vi "magnet_controller.vi"(1 "Arguments":string, 2 "Command":T1(ring)=enum."Hold", 3 "Direction":enum16{"X", "Y", "Z"}(ring)=enum."Y") -> (0 "Response":string)   [LabVIEW 2021]
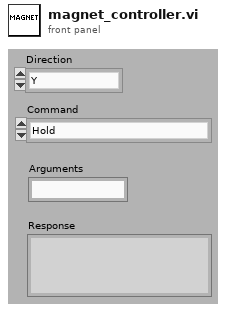
[diagram p1: front panel]
types:
  T1 = enum16{"Read State", "Hold", "Ramp to Set", "Ramp to Zero", "Read Switch Heater", "Switch Heater On", "Switch Heater Off", "Read Voltage", "Read Current", "Read Field", "Read Persistent Field", "Read Target Field", "Set Target Field", "Read Ramp Rate", "Set Ramp Rate"}
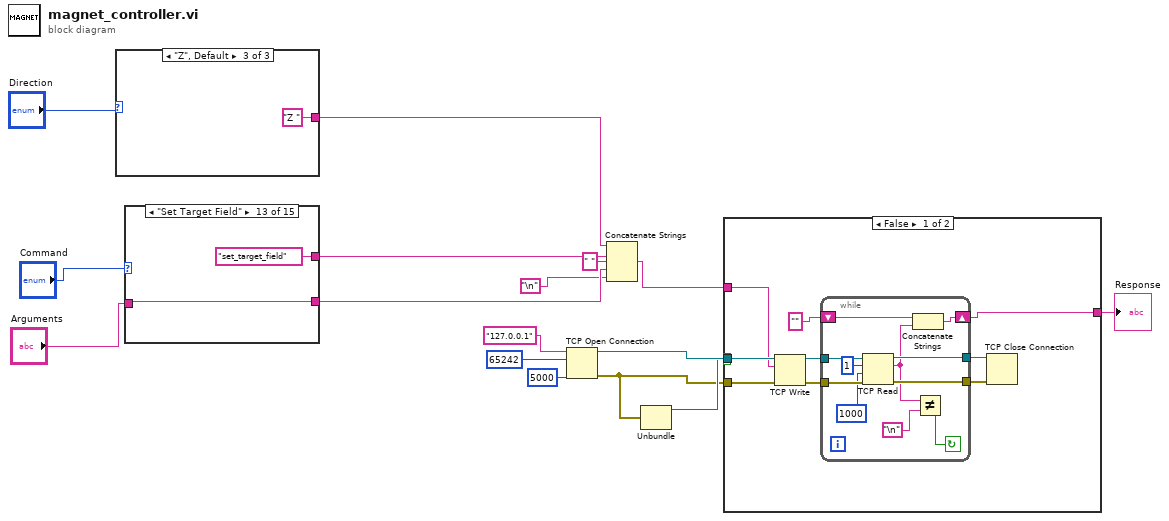
[diagram p0: block diagram]
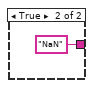
[diagram p2: hidden frame]
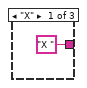
[diagram p3: hidden frame]
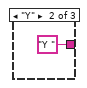
[diagram p4: hidden frame]
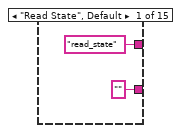
[diagram p5: hidden frame]
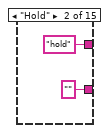
[diagram p6: hidden frame]
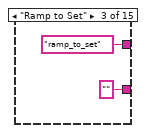
[diagram p7: hidden frame]
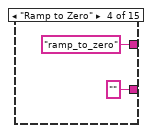
[diagram p8: hidden frame]
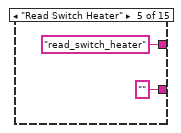
[diagram p9: hidden frame]
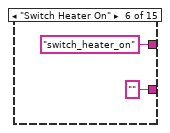
[diagram p10: hidden frame]
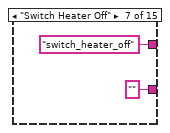
[diagram p11: hidden frame]
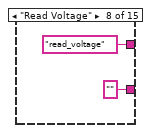
[diagram p12: hidden frame]
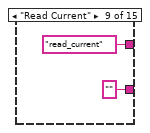
[diagram p13: hidden frame]
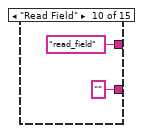
[diagram p14: hidden frame]
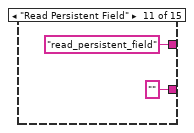
[diagram p15: hidden frame]
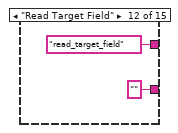
[diagram p16: hidden frame]
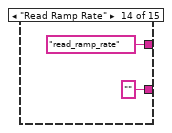
[diagram p17: hidden frame]
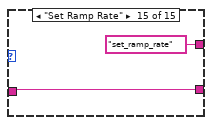
[diagram p18: hidden frame]
diagram:
  n1 = case shown="\"Z\", Default" "Direction" {
    tunnel: ["X " ("string") "Y " ("string") "Z " ("string")] -> w5
    frame "X" {
    }
    frame "Y" {
    }
    frame "Z", Default {
    }
  }
  n2 = case shown="\"Set Target Field\"" "Command" {
    tunnel: ["read_state" ("data in") "hold" ("data in") "ramp_to_set" ("data in") "ramp_to_zero" ("data in") "read_switch_heater" ("data in") "switch_heater_on" ("data in") "switch_heater_off" ("data in") "read_voltage" ("data in") "read_current" ("data in") "read_field" ("data in") "read_persistent_field" ("data in") "read_target_field" ("data in") "set_target_field" ("data in") "read_ramp_rate" ("data in") "set_ramp_rate" ("data in")] -> w12
    tunnel: ["" ("Arguments") "" ("Arguments") "" ("Arguments") "" ("Arguments") "" ("Arguments") "" ("Arguments") "" ("Arguments") "" ("Arguments") "" ("Arguments") "" ("Arguments") "" ("Arguments") "" ("Arguments") w44 "" ("Arguments") w48] -> w9
    tunnel: "Arguments" -> [_ _ _ _ _ _ _ _ _ _ _ _ w44 _ w48]
    frame "Read State", Default {
    }
    frame "Hold" {
    }
    frame "Ramp to Set" {
    }
    frame "Ramp to Zero" {
    }
    frame "Read Switch Heater" {
    }
    frame "Switch Heater On" {
    }
    frame "Switch Heater Off" {
    }
    frame "Read Voltage" {
    }
    frame "Read Current" {
    }
    frame "Read Field" {
    }
    frame "Read Persistent Field" {
    }
    frame "Read Target Field" {
    }
    frame "Set Target Field" {
    }
    frame "Read Ramp Rate" {
    }
    frame "Set Ramp Rate" {
    }
  }
  n3 = TCP Open Connection(address="127.0.0.1", remote port or service name=u16 65242, timeout ms (60000)=5000) -> (connection ID=w14:refnum<k5>, error out=w2:errorcluster)  [unwired: 2 in]
  n4 = Concatenate Strings(w5, w12, " " ("string"), w9, "\n") -> (w13:string)
  n5 = Unbundle(w2) -> ("status"=w3:bool)  [unwired: 2 out]
  n6 = case shown="False" w3 {
    tunnel: w14 -> [w58 _]
    tunnel: w2 -> [w57 _]
    tunnel: w13 -> [w51 _]
    tunnel: [w50 "NaN" ("string")] -> w4
    frame False {
      n7 = TCP Write(connection ID=w58, data in=w51, error in (no error)=w57) -> (connection ID out=w55:refnum<k5>, error out=w56:errorcluster)  [unwired: 1 in, 1 out]
      n8 = while {
        tunnel: w56 -> [w69]
        tunnel: w55 -> [w68]
        tunnel: [w67] -> w54
        tunnel: [w66] -> w53
        shift-right: [w62] -> w50
        shift-left: "" ("string") -> [w63]
        stop <- w61 continue-if-true
        n9 = TCP Read(connection ID=w68, bytes to read=1, error in (no error)=w69, 9:1000 ("timeout ms (25000)")) -> (connection ID out=w66:refnum<k5>, data out=w60:string, error out=w67:errorcluster)  [unwired: 1 in]
        n10 = Concatenate Strings(w63, w60) -> (w62:string)
        n11 = Not Equal?(x=w60, y="\n") -> (x != y?=w61:bool)
      }
      n12 = TCP Close Connection(connection ID=w53, error in (no error)=w54) -> ()  [unwired: 1 in, 2 out]
    }
    frame True {
    }
  }
  "Response" <- w4
